vi "x502_close.vi"(1 "error in (no error)":errorcluster, 2 "x502 in":refnum<k24>) -> (0 "error out (no error)":errorcluster)   [LabVIEW 2010]
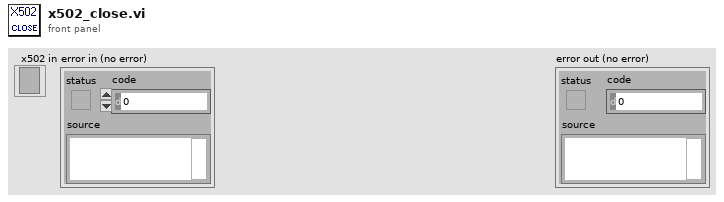
[diagram p1: front panel]
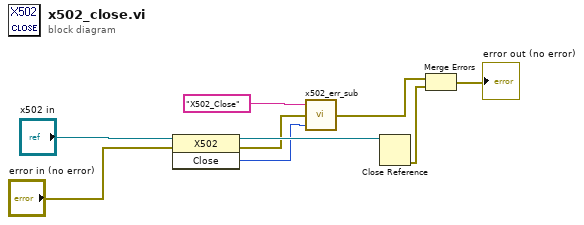
[diagram p0: block diagram]
diagram:
  n1 = invoke class="X502" method="Close"(reference="x502 in", error in="error in (no error)") -> (reference out=w9:refnum<k24>, error out=w7:errorcluster, "Close"=w6:i32)  [unwired: 1 in]
  n2 = call "x502_err_sub.vi"("Error code"=w6, "error in (no error)"=w7, "Error descr"="X502_Close") -> ("error out"=w4:errorcluster)
  n3 = Close Reference(reference=w9) -> (error out=w5:errorcluster)  [unwired: 1 in]
  n4 = Merge Errors(w4, w5) -> (→"error out (no error)":errorcluster)
